vi "Read Assembly config file.vi"(8 "error in (no error)":errorcluster, 11 "file (use dialog)":path=path "C:/git/fmussi_Ethernet-IP-Custom-Device/Tests/TestAssemblyConfig.csv") -> (0 "error out":errorcluster, 3 "Config":T1[](array[typedef]))   [LabVIEW 2023]
uses:
  Source/EIP Attribute Tag Configuration.ctl
  Source/EIP Attribute Direction.ctl
  <vilib>/Utility/file.llb/Read Delimited Spreadsheet (string).vi
  Source/Ethernet IP Custom Device Custom Device.lvlib
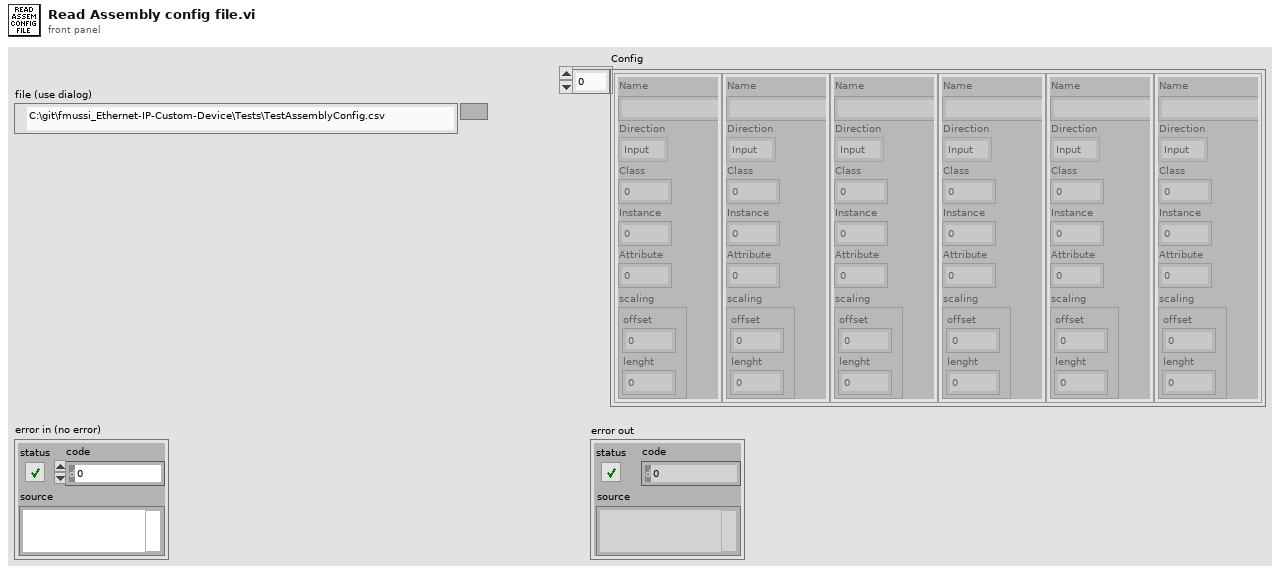
[diagram p1: front panel]
types:
  T1 = typedef "Ethernet IP Custom Device Custom Device.lvlib/EIP Attribute Tag Configuration.ctl" = cluster{"Name":string, "Direction":T2, "Class":i32, "Instance":u32, "Attribute":i32, "scaling":cluster{"offset":u32, "lenght":u32}}
  T2 = typedef "Ethernet IP Custom Device Custom Device.lvlib/EIP Attribute Direction.ctl" = enum16{"Input", "Output"}
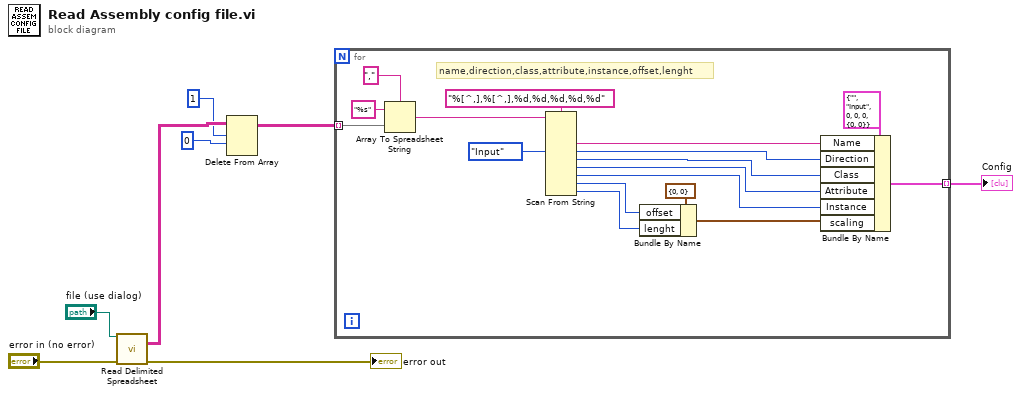
[diagram p0: block diagram]
diagram:
  n1 = call-poly <vilib>:"Read Delimited Spreadsheet.vi"("file path (dialog if empty)"="file (use dialog)", "error in (no error)"="error in (no error)") -> ("all rows"=w4:string[][], "error out"=→"error out":errorcluster)  [unwired: 8 in, 4 out]
  n2 = Delete From Array(array=w4, length=1 ("index (row)"), index (row)=0) -> (array with subset deleted=w3:string[][])  [unwired: 1 in, 1 out]
  n3 = for {
    tunnel: w3 -> [w25] mode=indexing
    tunnel: [w16] -> w5 mode=indexing
    # "name,direction,class,attribute,instance,offset,lenght"
    n4 = Array To Spreadsheet String(delimiter (Tab)=",", array=w25, 3:"%s" ("format string")) -> (spreadsheet string=w22:string)
    n5 = Scan From String(format string="%[^,],%[^,],%d,%d,%d,%d,%d", input string=w22, default 2=EIP_Attribute_Direction."Input" ("direction")) -> (output 1=w18:string, output 2=w17:T2, output 3=w15:i32, output 4=w14:i32, output 5=w13:i32, output 6=w11:i32, output 7=w10:i32)  [unwired: 8 in, 3 out]
    n6 = Bundle By Name(cluster=cluster{"offset":u32, "lenght":u32} {"offset"=0, "lenght"=0} ("scaling"), "offset"=w11, "lenght"=w10) -> (w9:cluster{"offset":u32, "lenght":u32})
    n7 = Bundle By Name(cluster=T1 {"Name"="", "Direction"=enum."Input", "Class"=0, "Instance"=0, "Attribute"=0, "scaling"={"offset"=0, "lenght"=0}} ("Config"), "Name"=w18, "Direction"=w17, "Class"=w15, "Attribute"=w14, "Instance"=w13, "scaling"=w9) -> (w16:T1)
  }
  "Config" <- w5
